vi "Periodic Tasks.vi"(8 "error in":errorcluster) -> ()   [LabVIEW 2015]
doc: "This VI runs in parallel to other tasks. It can contain as many user-defined periodic loops as you need. These can carry out PID or other sorts of timed response."
uses:
  <vilib>/Rock Robotics/WPI/Utilities/WPI_GetSetVariantRefNum.vi
  Robot Global Data.vi
  <vilib>/Rock Robotics/Network Tables/NT Write Number.vi
  navX Library v2/navX Library v2.lvlib
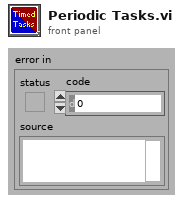
[diagram p1: front panel]
types:
  T1 = typedef "navX Library v2.lvlib/Z900_navX_DeviceTypeDef.ctl" = cluster{"Interface":cluster{"Protocol":T2, "Update Rate (4Hz-60Hz)":u8, "navX Open TypeDef":variant}, "Notify Packet":refnum<notifier>, "Loop VI Refnum":refnum<vi>, "Ready to Close Occurrence Refnum":refnum<k4>}
  T2 = typedef "navX Library v2.lvlib/Z900_navX_ProtocolTypeDef.ctl" = enum16{"SERIAL", "I2C", "SPI"}
  T3 = typedef "WPI_EncoderDevRef.ctl" = cluster{"DevStatus":errorcluster, "EncoderIndex":T4, "CounterIndex":T5, "DistancePerCount":dbl, "Decoding Type":T6}
  T4 = typedef "FPGA_EncoderIdx.ctl" = enum8{"Enc 0", "Enc 1", "Enc 2", "Enc 3", "Enc 4", "Enc 5", "Enc 6", "Enc 7", "Invalid"}
  T5 = typedef "FPGA_CounterCtrSystemIndex.ctl" = enum8{"Ctr 0", "Ctr 1", "Ctr 2", "Ctr 3", "Ctr 4", "Ctr 5", "Ctr 6", "Ctr 7", "Invalid"}
  T6 = typedef "WPI_EncoderType.ctl" = enum16{"1x", "2x", "4x"}
  T7 = cluster{"Yaw":dbl, "Roll":dbl, "Pitch":dbl, "Heading":dbl, "Fused Heading":dbl}
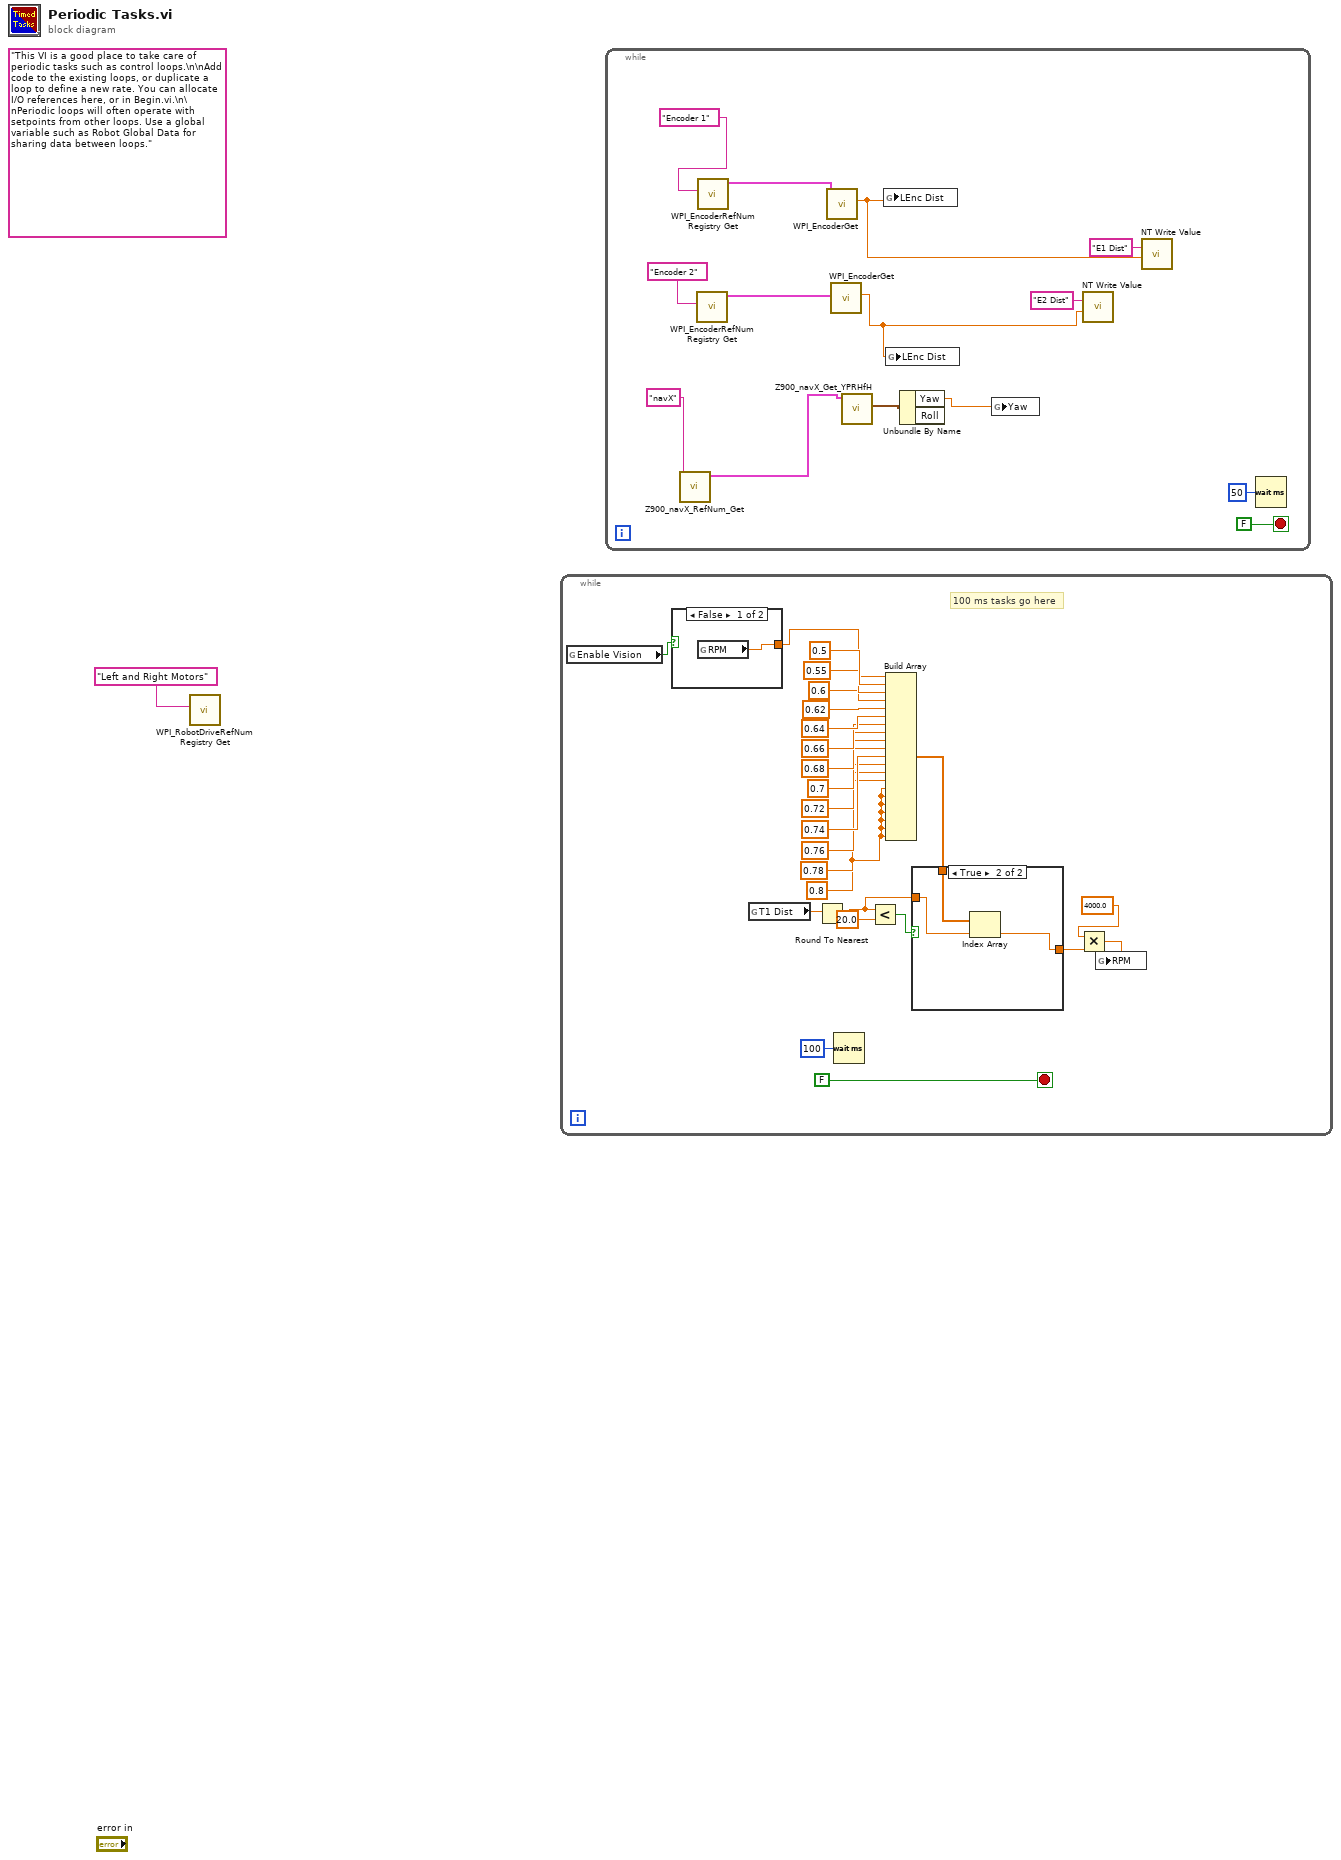
[diagram p0: block diagram]
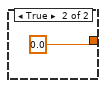
[diagram p2: hidden frame]
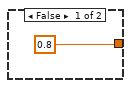
[diagram p3: hidden frame]
diagram:
  (unwired) "This VI is a good place to take care of periodic tasks such as control loops.\n\nAdd code to the existing loops, or duplicate a loop to define a new rate. You can allocate I/O references here, or in Begin.vi.\n\nPeriodic loops will often operate with setpoints from other loops. Use a global variable such as Robot Global Data for sharing data between loops."
  n1 = call <vilib>:"WPI_RobotDriveRefNum Registry Get.vi"("refnum name"="Left and Right Motors") -> ()  [unwired: 1 in, 10 out]
  n2 = while {
    stop <- FALSE stop-if-true
    w11 = 0.8 ("element")
    # "100 ms tasks go here"
    n3 = global read "Robot Global Data.vi" "Enable Vision"() -> (w6:bool)
    n4 = case shown="False" w6 {
      tunnel: [w27 0.0 ("element")] -> w5
      frame False {
        n5 = global read "Robot Global Data.vi" "RPM"() -> (w27:dbl)
      }
      frame True {
      }
    }
    n6 = global read "Robot Global Data.vi" "T1 Dist"() -> (w24:dbl)
    n7 = Round To Nearest(number=w24) -> (nearest integer value=w7:dbl)
    n8 = Wait (ms)(milliseconds to wait=u32 100) -> ()  [unwired: 1 out]
    n9 = Less?(x=w7, y=20.0) -> (x < y?=w9:bool)
    n10 = Build Array(w5, 0.5 ("element"), 0.55 ("element"), 0.6 ("element"), 0.62 ("element"), 0.64 ("element"), 0.66 ("element"), 0.68 ("element"), 0.7 ("element"), 0.72 ("element"), 0.74 ("element"), 0.76 ("element"), 0.78 ("element"), w11, w11, w11, w11, w11, w11, w11, w11) -> (w8:dbl[])
    n11 = case shown="True" w9 {
      tunnel: w8 -> [_ w31]
      tunnel: [0.8 w30] -> w3
      tunnel: w7 -> [_ w32]
      frame False {
      }
      frame True {
        n12 = Index Array(array=w31, index=w32) -> (element=w30:dbl)
      }
    }
    n13 = Multiply(x=4000.0, y=w3) -> (x*y=w2:dbl)
    n14 = global write "Robot Global Data.vi" "RPM"(w2) -> ()
  }
  n15 = while {
    stop <- FALSE stop-if-true
    n16 = call "Z900_navX_RefNum_Get.vi"("refnum name"="navX") -> ("navX Device"=w33:T1)  [unwired: 9 in, 1 out]
    n17 = call <vilib>:"WPI_EncoderRefNum Registry Get.vi"("refnum name"="Encoder 2") -> ("EncoderDevRef"=w35:T3)  [unwired: 9 in, 1 out]
    n18 = call <vilib>:"WPI_EncoderRefNum Registry Get.vi"("refnum name"="Encoder 1") -> ("EncoderDevRef"=w34:T3)  [unwired: 9 in, 1 out]
    n19 = call <vilib>:"WPI_EncoderGet.vi"("EncoderDevRef"=w34) -> ("Distance"=w37:dbl)  [unwired: 5 in, 5 out]
    n20 = call <vilib>:"WPI_EncoderGet.vi"("EncoderDevRef"=w35) -> ("Distance"=w36:dbl)  [unwired: 5 in, 5 out]
    n21 = call "Z900_navX_Get_YPRHfH.vi"("navX Device"=w33) -> ("YRPHfH"=w41:T7)  [unwired: 7 in, 3 out]
    n22 = global write "Robot Global Data.vi" "LEnc Dist"(w37) -> ()
    n23 = global write "Robot Global Data.vi" "LEnc Dist"(w36) -> ()
    n24 = Unbundle By Name(w41) -> ("Yaw"=w40:dbl)  [unwired: 1 out]
    n25 = global write "Robot Global Data.vi" "Yaw"(w40) -> ()
    n26 = call-poly <vilib>:"NT Write Value.vi"("Numeric"=w36, "Name"="E2 Dist") -> ()  [unwired: 9 in, 1 out]
    n27 = call-poly <vilib>:"NT Write Value.vi"("Numeric"=w37, "Name"="E1 Dist") -> ()  [unwired: 9 in, 1 out]
    n28 = Wait (ms)(milliseconds to wait=u32 50) -> ()  [unwired: 1 out]
  }
